vi "GetGantryPosition.vi"(8 "error in (no error)":errorcluster, 10 "Controller In":refnum<k24>) -> (0 "error out":errorcluster, 1 "Position Y":dbl, 2 "Position X":dbl, 3 "controller out":refnum<k24>, 4 "Position U":dbl, 5 "Position_XYZ":string, 6 "Position Z":dbl)   [LabVIEW 2021]
uses:
  C:/Users/TTUHEP/Documents/LabVIEW/Other Models/2010/Bin/Aerotech.A3200.dll
  Other Models/2010/Bin/Aerotech.A3200.dll
panel:
  out "Program Position U":dbl
  out "Velocity U":dbl
  out "Program Position Z":dbl
  out "Velocity Z":dbl
  out "Program Position Y":dbl
  out "Velocity Y":dbl
  out "Program Position X":dbl
  out "Velocity X":dbl format="%#.5g"
  # "Get position of gantry head (GH). Units of X & Y are in mm."
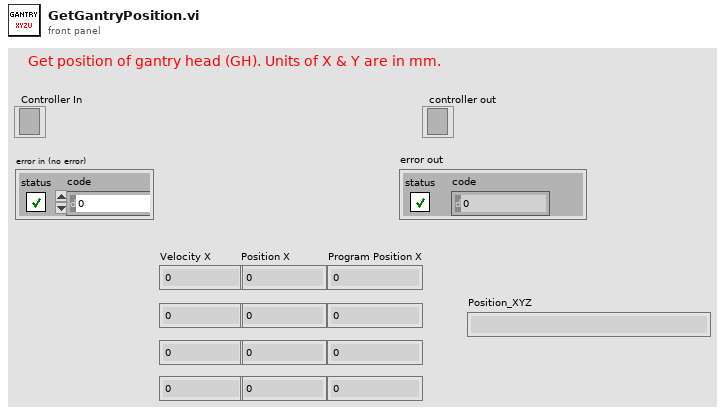
[diagram p1: front panel]
types:
  T1 = typedef "ControllerDiagPacket.ctl" = cluster{"Number of Diag Packets":i32, "Axes":T2[], "error":errorcluster}
  T2 = typedef "AxisDiagPacket.ctl" = cluster{"Axis Name":string, "Analog Input 0":dbl, "Analog Input 1":dbl, "Axis Fault (num)":i32, "Axis Fault (str)":string, "Axis Fault (bits)":cluster{"AmplifierFault":bool, "AmplifierTemperatureFault":bool, "CcwEndOfTravelLimitFault":bool, "CcwSoftwareLimitFault":bool, "CommunicationLostFault":bool, "CwEndOfTravelLimitFault":bool, "CwSoftwareLimitFault":bool, "EmergencyStopFault":bool, "EncoderFault":bool, "ExternalFault":bool, "FeedbackScalingFault":bool, "GantryMisalignFault ":bool, "HallSensorFault":bool, "InPositionTimeoutFault":bool, "InternalFault":bool, "MarkerSearchFault":bool, "MaxVelocityCommandFault":bool, "MissedInterruptFault":bool, "MotorTemperatureFault":bool, "None":bool, "OverCurrentFault":bool, "PositionErrorFault":bool, "PositionFeedbackFault":bool, "PowerSupplyFault":bool, "ProbeInputFault":bool, "SafeZoneFault":bool, "VelocityErrorFault":bool, "VelocityFeedbackFault":bool, "VoltageClampFault":bool}, "Axis Status (num)":i32, "Axis Status (str)":string, "Axis Status (bits)":cluster{"BacklashActive":bool, "CalibrationEnabled1D":bool, "CalibrationEnabled2D":bool, "CommandValid":bool, "DriveAbortPending":bool, "DrivePending":bool, "Enabling":bool, "GainMappingEnabled":bool, "GantryAligned":bool, "GantryRealigning":bool, "Homed":bool, "Homing":bool, "IFOVEnabled":bool, "JogGenerating":bool, "Jogging":bool, "JoystickControl":bool, "MasterSlaveControl":bool, "MotionBlocked":bool, "MotionClamped":bool, "MoveDone":bool, "None":bool, "NotVirtual":bool, "Profiling":bool, "Stability0":bool, "Stability1":bool, "TrajectoryFiltering":bool, "WaitDone":bool}, "Current Command":sgl, "Current Error":sgl, "Current Feedback":sgl, "Digital Inputs":i32, "Digital Outputs":i32, "Drive Status":i32, "Drive Status (str)":string, "Drive Status (bits)":cluster{"AccelerationPhase":bool, "AutofocusActive":bool, "BrakeOutput":bool, "CcwEndOfTravelLimitInput":bool, "CosineEncoderError":bool, "CurrentClamp":bool, "CwEndOfTravelLimitInput":bool, "DecelerationPhase":bool, "DualLoopActive":bool, "EmergencyStopInput":bool, "Enabled":bool, "EncoderClipping":bool, "GalvoCalibrationEnabled":bool, "GalvoPowerCorrection":bool, "HallAInput":bool, "HallBInput":bool, "HallCInput":bool, "HighResolutionMode":bool, "HomeLimitInput":bool, "InPosition":bool, "InPosition2":bool, "MarkerInput":bool, "MarkerLatch":bool, "MoveActive":bool, "NoMotorSupply":bool, "None":bool, "PowerLimiting":bool, "ProgrammingFlash":bool, "ProgrammingMXH":bool, "PSOHaltLatch":bool, "ServoControl":bool, "SineEncoderError":bool}, "Position Feedback Auxiliary":dbl, "Position Command":dbl, "Position Error":dbl, "Position Feedback":dbl, "Program Position Command":dbl, "Program Position Error":dbl, "Program Position Feedback":dbl, "Velocity Command":dbl, "Velocity Error":dbl, "Velocity Feedback":dbl}
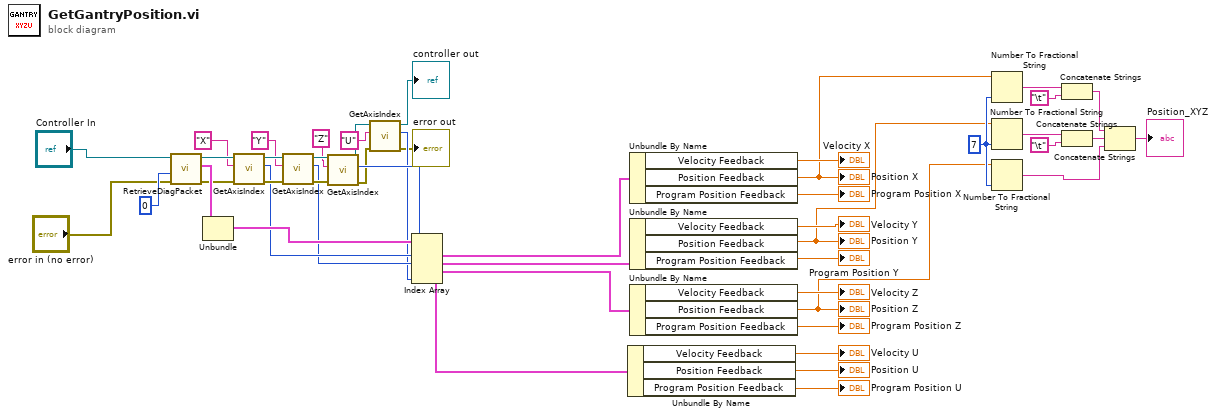
[diagram p0: block diagram]
diagram:
  w15 = i16 7 ("precision (6)")
  n1 = call "RetrieveDiagPacket.vi"("error in (no error)"="error in (no error)", "axisMask"=0, "Controller In"="Controller In") -> ("error out"=w47:errorcluster, "ControllerDiagPacket"=w48:T1, "Controller Out"=w46:refnum<k24>)  [unwired: 6 in]
  n2 = Unbundle(w48) -> ("Axes"=w39:T2[])  [unwired: 2 out]
  n3 = call "GetAxisIndex.vi"("error in (no error)"=w47, "axis name"="X", "controller in"=w46) -> ("error out"=w43:errorcluster, "axis index"=w38:i32, "controller out"=w45:refnum<k24>)  [unwired: 6 in]
  n4 = call "GetAxisIndex.vi"("error in (no error)"=w43, "axis name"="Y", "controller in"=w45) -> ("error out"=w42:errorcluster, "axis index"=w37:i32, "controller out"=w44:refnum<k24>)  [unwired: 6 in]
  n5 = call "GetAxisIndex.vi"("error in (no error)"=w42, "axis name"="Z", "controller in"=w44) -> ("error out"=w20:errorcluster, "axis index"=w36:i32, "controller out"=w27:refnum<k24>)  [unwired: 6 in]
  n6 = call "GetAxisIndex.vi"("error in (no error)"=w20, "axis name"="U", "controller in"=w27) -> ("error out"=→"error out":errorcluster, "axis index"=w25:i32, "controller out"=→"controller out":refnum<k24>)  [unwired: 6 in]
  n7 = Index Array(array=w39, index #1=w38, index #2=w37, index #3=w36, index #4=w25) -> (element #1=w34:T2, element #2=w32:T2, element #3=w33:T2, element #4=w24:T2)
  n8 = Unbundle By Name(w24) -> ("Velocity Feedback"=→"Velocity U":dbl, "Position Feedback"=→"Position U":dbl, "Program Position Feedback"=→"Program Position U":dbl)
  n9 = Unbundle By Name(w34) -> ("Velocity Feedback"=→"Velocity X":dbl, "Position Feedback"=w3:dbl, "Program Position Feedback"=→"Program Position X":dbl)
  "Position X" <- w3
  n10 = Unbundle By Name(w32) -> ("Velocity Feedback"=→"Velocity Y":dbl, "Position Feedback"=w2:dbl, "Program Position Feedback"=→"Program Position Y":dbl)
  "Position Y" <- w2
  n11 = Unbundle By Name(w33) -> ("Velocity Feedback"=→"Velocity Z":dbl, "Position Feedback"=w1:dbl, "Program Position Feedback"=→"Program Position Z":dbl)
  "Position Z" <- w1
  n12 = Number To Fractional String(number=w3, precision (6)=w15) -> (F-format string=w14:string)  [unwired: 2 in]
  n13 = Number To Fractional String(number=w2, precision (6)=w15) -> (F-format string=w11:string)  [unwired: 2 in]
  n14 = Number To Fractional String(number=w1, precision (6)=w15) -> (F-format string=w7:string)  [unwired: 2 in]
  n15 = Concatenate Strings(w14, "\t") -> (w10:string)
  n16 = Concatenate Strings(w11, "\t") -> (w9:string)
  n17 = Concatenate Strings(w10, w9, w7) -> (→"Position_XYZ":string)
